vi "ShooterPneumatics(SubVI).vi"(10 "Past Input Angle":bool, 11 "Angle":bool) -> (3 "New Input Angle":bool)   [LabVIEW 2017]
uses:
  <vilib>/Rock Robotics/WPI/Solenoid/WPI_SolenoidValue.ctl
  <vilib>/Rock Robotics/WPI/Solenoid/WPI_SolenoidSetEnum.vi
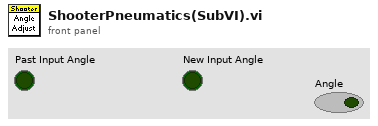
[diagram p1: front panel]
types:
  T1 = typedef "WPI_SolenoidValue.ctl" = enum16{"Off", "On", "Forward", "Reverse"}
  T2 = typedef "WPI_SolenoidDevRef.ctl" = cluster{"DevStatus":errorcluster, "Pneumatics Control Module":u8, "Forward Solenoid Channel":T3, "Reverse Solenoid Channel":T3}
  T3 = typedef "WPI_SolenoidChannel.ctl" = enum8{"Solenoid 0", "Solenoid 1", "Solenoid 2", "Solenoid 3", "Solenoid 4", "Solenoid 5", "Solenoid 6", "Solenoid 7", "Invalid"}
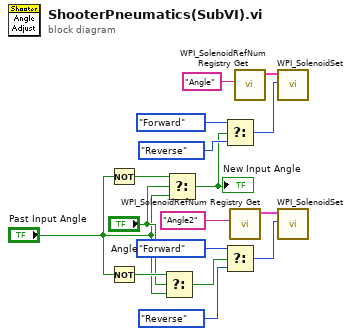
[diagram p0: block diagram]
diagram:
  n1 = Not(x="Past Input Angle") -> (.not. x?=w10:bool)
  n2 = Not(x="Past Input Angle") -> (.not. x?=w11:bool)
  n3 = Select(t=w11, s="Angle", f="Past Input Angle") -> (s? t:f=w3:bool)
  n4 = Select(t=w10, s="Angle", f="Past Input Angle") -> (s? t:f=w4:bool)
  "New Input Angle" <- w4
  n5 = Select(t=WPI_SolenoidValue."Forward" ("Value"), s=w4, f=WPI_SolenoidValue."Reverse" ("Value")) -> (s? t:f=w9:T1)
  n6 = Select(t=WPI_SolenoidValue."Forward" ("Value"), s=w3, f=WPI_SolenoidValue."Reverse" ("Value")) -> (s? t:f=w12:T1)
  n7 = call <vilib>:"WPI_SolenoidRefNum Registry Get.vi"("refnum name"="Angle2") -> ("SolenoidDevRef"=w15:T2)  [unwired: 9 in, 1 out]
  n8 = call <vilib>:"WPI_SolenoidRefNum Registry Get.vi"("refnum name"="Angle") -> ("SolenoidDevRef"=w6:T2)  [unwired: 9 in, 1 out]
  n9 = call-poly <vilib>:"WPI_SolenoidSet.vi"("Value"=w9, "SolenoidDevRef"=w6) -> ()  [unwired: 8 in, 2 out]
  n10 = call-poly <vilib>:"WPI_SolenoidSet.vi"("Value"=w12, "SolenoidDevRef"=w15) -> ()  [unwired: 8 in, 2 out]
